vi "Vision Shooter Lineup.vi"(4 "X axis value":dbl=20.0 format="%#_13g", 5 "X axis value 2":dbl=-20.0, 9 "Intake":dbl=-100.0) -> ()   [LabVIEW 2015]
uses:
  Robot Global Data.vi
panel:
  in  "Distance Type":enum16{"SONAR", "VISION", "BOTH"}(ring)
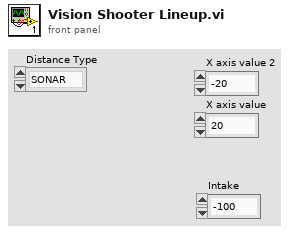
[diagram p1: front panel]
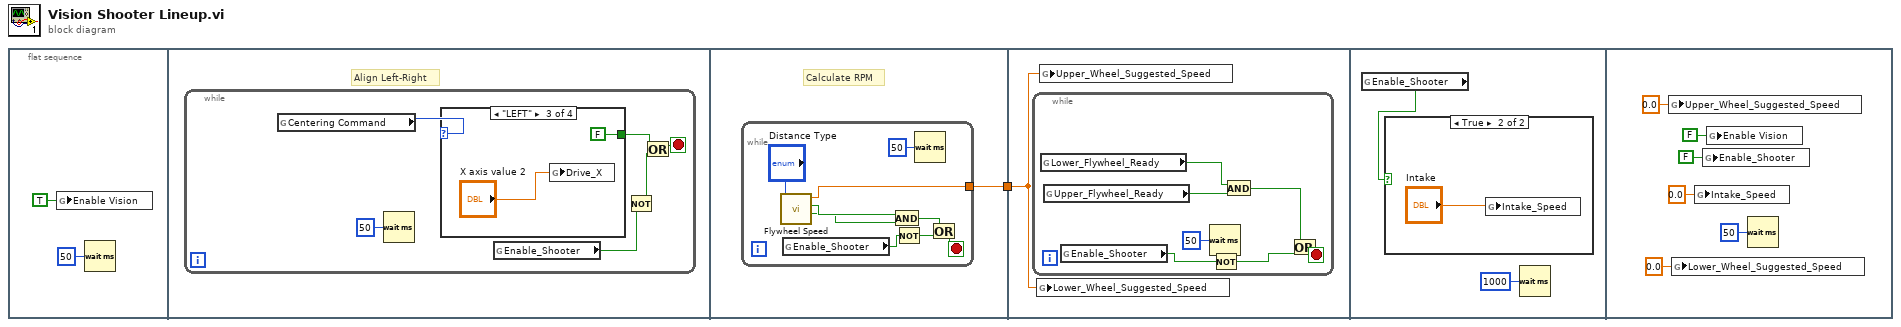
[diagram p0: block diagram]
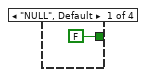
[diagram p2: hidden frame]
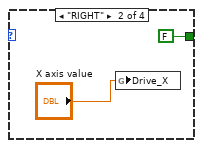
[diagram p3: hidden frame]
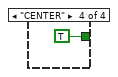
[diagram p4: hidden frame]
diagram:
  n1 = flat-sequence {
    tunnel: [w16] -> w1
    tunnel: w1 -> [w26]
    frame #0 {
      n2 = global write "Robot Global Data.vi" "Enable Vision"(TRUE ("Enable Vision")) -> ()
      n3 = Wait (ms)(milliseconds to wait=u32 50) -> ()  [unwired: 1 out]
    }
    frame #1 {
      # "Align Left-Right"
      n4 = while {
        stop <- w6 stop-if-true
        n5 = global read "Robot Global Data.vi" "Centering Command"() -> (w8:enum16{"NULL", "RIGHT", "LEFT", "CENTER"})
        n6 = Wait (ms)(milliseconds to wait=u32 50) -> ()  [unwired: 1 out]
        n7 = case shown="\"LEFT\"" w8 {
          tunnel: [FALSE FALSE FALSE TRUE] -> w9
          frame "NULL", Default {
          }
          frame "RIGHT" {
            n8 = global write "Robot Global Data.vi" "Drive_X"("X axis value") -> ()
          }
          frame "LEFT" {
            n9 = global write "Robot Global Data.vi" "Drive_X"("X axis value 2") -> ()
          }
          frame "CENTER" {
          }
        }
        n10 = global read "Robot Global Data.vi" "Enable_Shooter"() -> (w5:bool)
        n11 = Not(x=w5) -> (.not. x?=w4:bool)
        n12 = Or(x=w9, y=w4) -> (x .or. y?=w6:bool)
      }
    }
    frame #2 {
      # "Calculate RPM"
      n13 = while {
        tunnel: [w22] -> w16
        stop <- w19 stop-if-true
        n14 = call "Flywheel Speed.vi"("Distance Type"="Distance Type") -> ("Calculation_Ready"=w23:bool, "In_Range"=w24:bool, "Suggested Speed"=w22:dbl)  [unwired: 8 in]
        n15 = global read "Robot Global Data.vi" "Enable_Shooter"() -> (w18:bool)
        n16 = And(x=w24, y=w23) -> (x .and. y?=w25:bool)
        n17 = Not(x=w18) -> (.not. x?=w17:bool)
        n18 = Wait (ms)(milliseconds to wait=u32 50) -> ()  [unwired: 1 out]
        n19 = Or(x=w25, y=w17) -> (x .or. y?=w19:bool)
      }
    }
    frame #3 {
      n20 = while {
        stop <- w29 stop-if-true
        n21 = global read "Robot Global Data.vi" "Lower_Flywheel_Ready"() -> (w32:bool)
        n22 = global read "Robot Global Data.vi" "Upper_Flywheel_Ready"() -> (w33:bool)
        n23 = global read "Robot Global Data.vi" "Enable_Shooter"() -> (w28:bool)
        n24 = Wait (ms)(milliseconds to wait=u32 50) -> ()  [unwired: 1 out]
        n25 = Not(x=w28) -> (.not. x?=w27:bool)
        n26 = And(x=w32, y=w33) -> (x .and. y?=w31:bool)
        n27 = Or(x=w31, y=w27) -> (x .or. y?=w29:bool)
      }
      n28 = global write "Robot Global Data.vi" "Lower_Wheel_Suggested_Speed"(w26) -> ()
      n29 = global write "Robot Global Data.vi" "Upper_Wheel_Suggested_Speed"(w26) -> ()
    }
    frame #4 {
      n30 = global read "Robot Global Data.vi" "Enable_Shooter"() -> (w34:bool)
      n31 = case shown="True" w34 {
        frame False {
        }
        frame True {
          n32 = global write "Robot Global Data.vi" "Intake_Speed"("Intake") -> ()
        }
      }
      n33 = Wait (ms)(milliseconds to wait=u32 1000) -> ()  [unwired: 1 out]
    }
    frame #5 {
      n34 = global write "Robot Global Data.vi" "Upper_Wheel_Suggested_Speed"(0.0 ("Upper_Wheel_Suggested_Speed")) -> ()
      n35 = global write "Robot Global Data.vi" "Lower_Wheel_Suggested_Speed"(0.0 ("Lower_Wheel_Suggested_Speed")) -> ()
      n36 = global write "Robot Global Data.vi" "Intake_Speed"(0.0 ("Intake_Speed")) -> ()
      n37 = global write "Robot Global Data.vi" "Enable_Shooter"(FALSE ("Enable_Shooter")) -> ()
      n38 = global write "Robot Global Data.vi" "Enable Vision"(FALSE ("Enable Vision")) -> ()
      n39 = Wait (ms)(milliseconds to wait=u32 50) -> ()  [unwired: 1 out]
    }
  }
